vi "pathplan.vi"() -> ()   [LabVIEW 2016]
panel:
  in  "当前位置":dbl[](array[numeric])
  in  "目标位置":dbl[](array[numeric])
  out "写入缓冲区":string
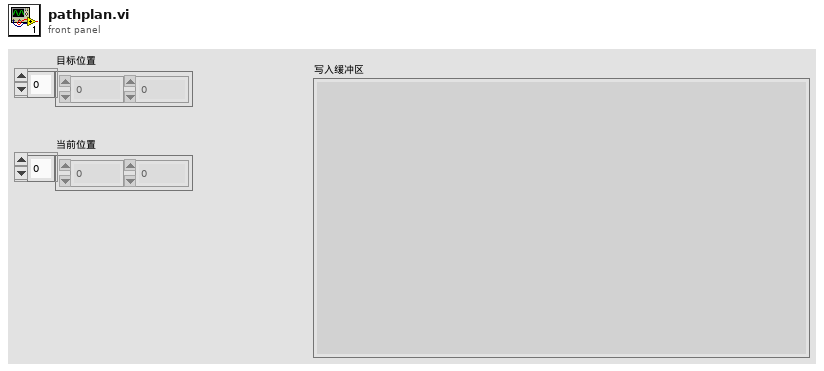
[diagram p1: front panel]
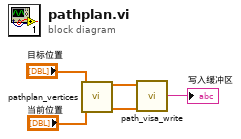
[diagram p0: block diagram]
diagram:
  n1 = call "pathplan_vertices.vi"("目标位置（x,y）"="目标位置", "当前位置"="当前位置") -> ("x"=w5:dbl[], "y"=w4:dbl[])  [unwired: 7 in]
  n2 = call "path_visa_write.vi"("y"=w4, "x"=w5) -> ("写入缓冲区"=→"写入缓冲区":string)  [unwired: 9 in]
